vi "Init Series Graph.vi"(6 "Z Scale.Marker Values[]":cluster{"Numeric":dbl, "Numeric":u32}[](array[cluster]), 7 "Graphs":T1, 8 "error in":errorcluster, 9 "Shots":u32, 10 "Image Size":cluster{"Rows":u32, "Cols":u32}, 11 "Series Graph in":refnum<class "Graph with Series View.lvclass">) -> (0 "error out":errorcluster, 3 "Series Graph out":refnum<class "Graph with Series View.lvclass">)   [LabVIEW 2025, in "Graph with Series View.lvclass"]
uses:
  Graph with Series View.lvclass
  Graph with Series View.lvclass/Graph with Series View.ctl
  Detail Graph/Graph with Section Views.lvclass
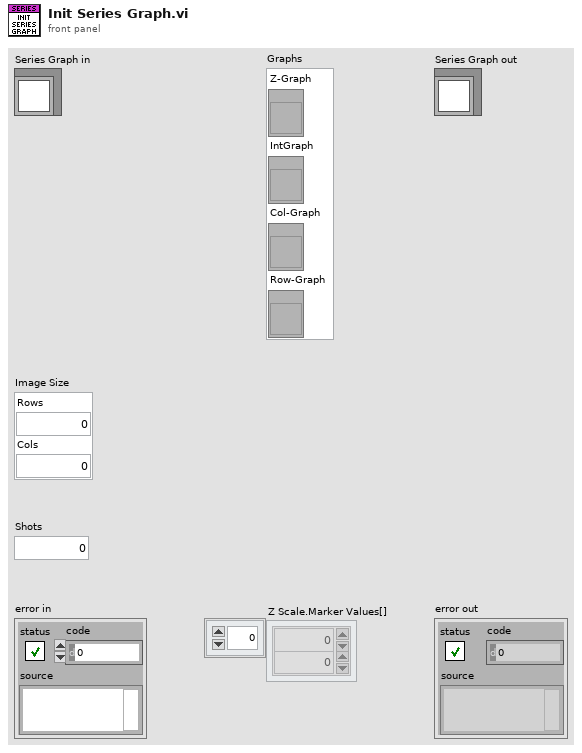
[diagram p1: front panel]
types:
  T1 = cluster{"Z-Graph":refnum<vi>, "IntGraph":refnum<vi>, "Col-Graph":refnum<vi>, "Row-Graph":refnum<vi>}
  T2 = cluster{"IntGraph":refnum<vi>, "Col-Graph":refnum<vi>, "Row-Graph":refnum<vi>}
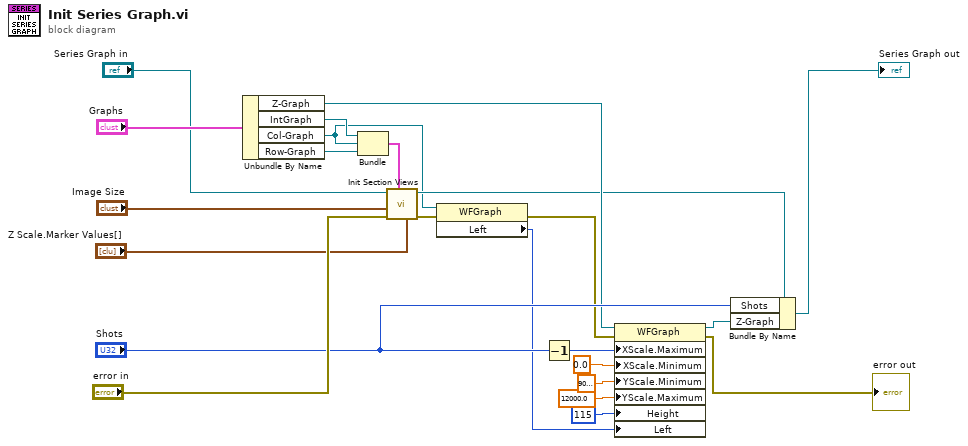
[diagram p0: block diagram]
diagram:
  n1 = Unbundle By Name("Graphs") -> ("Z-Graph"=w7:refnum<vi>, "IntGraph"=w3:refnum<vi>, "Col-Graph"=w1:refnum<vi>, "Row-Graph"=w9:refnum<vi>)
  n2 = Bundle("IntGraph"=w3, "Col-Graph"=w1, "Row-Graph"=w9) -> (w8:T2)  [unwired: 1 in]
  n3 = call "Init Section Views.vi"("Z Scale.Marker Values[]"="Z Scale.Marker Values[]", "Graphs"=w8, "error in"="error in", "Image Size"="Image Size", "Detail Graph.lvclass"="Series Graph in") -> ("error out"=w15:errorcluster, "Detail Graph out.lvclass"=w6:refnum<class "Graph with Series View.lvclass">)  [unwired: 5 in]
  n4 = property class="WFGraph"(reference=w1, error in=w15) -> (error out=w4:errorcluster, "Left"=w2:i32)  [unwired: 1 out]
  n5 = Decrement(x="Shots") -> (x-1=w10:u32)
  n6 = property class="WFGraph"(reference=w7, error in=w4, "XScale.Maximum"=w10, "XScale.Minimum"=0.0 ("X Scale.Range:Minimum"), "YScale.Minimum"=9000.0 ("Y Scale.Range:Minimum"), "YScale.Maximum"=12000.0 ("Y Scale.Range:Maximum"), "Height"=u32 115 ("Plot Area:Size:Height"), "Left"=w2) -> (reference out=w5:refnum<vi>, error out=→"error out":errorcluster)
  n7 = Bundle By Name(cluster=w6, "Shots"="Shots", "Z-Graph"=w5) -> (→"Series Graph out":refnum<class "Graph with Series View.lvclass">)
